vi "AddSingleSingle.vi"(7 "Priority":refnum<class "Action.lvclass">, 10 "Standard":refnum<class "Action.lvclass">, 11 "Stack in":refnum<class "Stack.lvclass">) -> (3 "Stack out":refnum<class "Stack.lvclass">)   [LabVIEW 2024, in "ActionStack.lvlib" / "Stack.lvclass"]
uses:
  Stack.lvclass
  Action/Action.lvclass
  Stack.lvclass/Stack.ctl
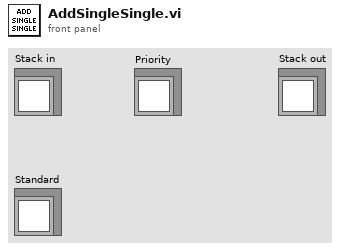
[diagram p1: front panel]
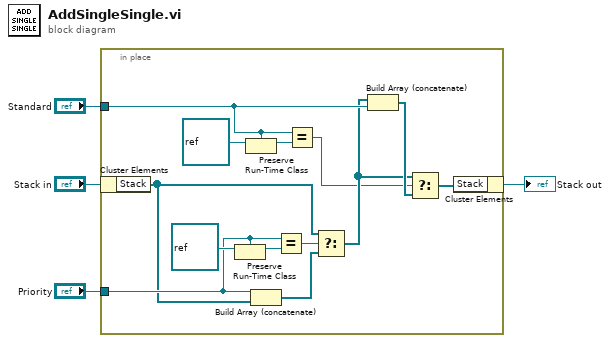
[diagram p0: block diagram]
diagram:
  n1 = in-place {
    in-place-border: "Priority" -> [w13]
    in-place-border: "Standard" -> [w10]
    n2 = in-place-cluster #1("Stack in") -> ("Stack"=w6:refnum<class "Action.lvclass">[])
    n3 = Preserve Run-Time Class(object in=refnum<class> refnum, 2:w13) -> (object out=w14:refnum<class "Action.lvclass">)  [unwired: 1 in, 1 out]
    n4 = Preserve Run-Time Class(object in=refnum<class> refnum, 2:w10) -> (object out=w16:refnum<class "Action.lvclass">)  [unwired: 1 in, 1 out]
    n5 = Build Array (concatenate)(w13, w6) -> (w11:refnum<class "Action.lvclass">[])
    n6 = Equal?(x=w13, y=w14) -> (x = y?=w12:bool)
    n7 = Equal?(x=w10, y=w16) -> (x = y?=w7:bool)
    n8 = Select(t=w6, s=w12, f=w11) -> (s? t:f=w8:refnum<class "Action.lvclass">[])
    n9 = Build Array (concatenate)(w8, w10) -> (w9:refnum<class "Action.lvclass">[])
    n10 = Select(t=w8, s=w7, f=w9) -> (s? t:f=w5:refnum<class "Action.lvclass">[])
    n11 = in-place-cluster #1("Stack"=w5) -> (→"Stack out":refnum<class "Stack.lvclass">)
  }
